vi "GetMessage.vi"(8 "entrée d'erreur":errorcluster caption="entrée d'erreur (pas d'erreur)", 11 "Message queue":refnum<queue>) -> (0 "sortie d'erreur":errorcluster, 1 "Data":variant, 2 "Message":string, 3 "Dup Message Queue":refnum<queue>)   [LabVIEW 2013, in "MessageQueues.lvlib"]
doc: "Ce VI permet la récupération d'un message en bas de pile, ainsi que sa donnée. Fonctionne en FIFO : First In First Out.\n\nEntrée :\nMessage queue : la pile concernée\nerror : entrée d'erreur\n\nSortie :\nDup Message Queue : Pile décrémenté\nMessage : Message récupéré en bas de pile\nData : Donnée lié au message du type variant.\nerro : sortie d'erreur."
uses:
  MessageQueues.lvlib
  Message Cluster.ctl
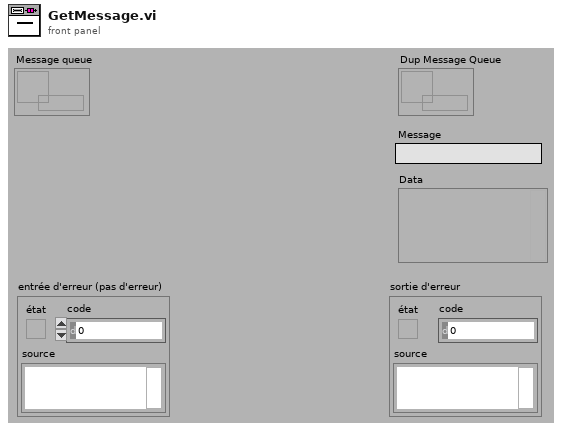
[diagram p1: front panel]
types:
  T1 = typedef "MessageQueues.lvlib/Message Cluster.ctl" = cluster{"Message":string, "Data":variant}
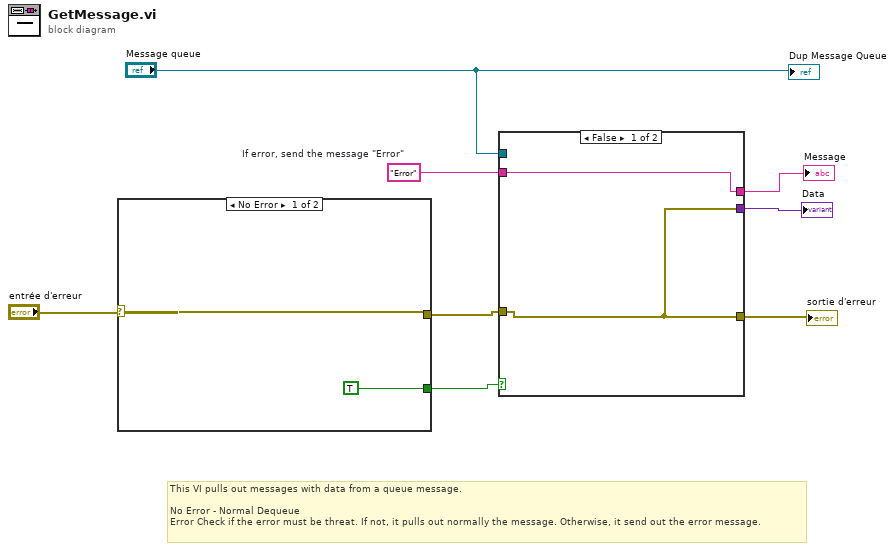
[diagram p0: block diagram]
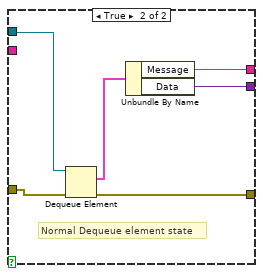
[diagram p2: hidden frame]
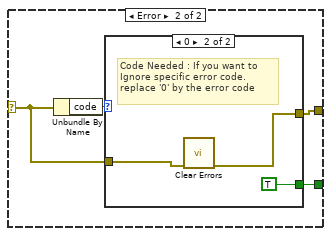
[diagram p3: hidden frame]
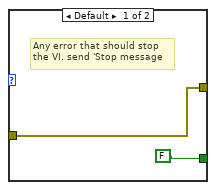
[diagram p4: hidden frame]
diagram:
  w5 = "Error"  # If error, send the message "Error"
  # "This VI pulls out messages with data from a queue message.\n\nNo Error - Normal Dequeue\nError Check if the error must be threat. If not, it pulls out normally the message. Otherwise, it send out the error message."
  n1 = case shown="No Error" "entrée d'erreur" {
    selector: "entrée d'erreur" -> [w9 w12]
    tunnel: [TRUE w14] -> w7
    tunnel: [w9 w11] -> w6
    frame No Error {
    }
    frame Error {
      n2 = Unbundle By Name(w12) -> ("code"=w13:i32)
      n3 = case shown="0" w13 {
        tunnel: [FALSE TRUE] -> w14
        tunnel: w12 -> [w15 w18]
        tunnel: [w15 w17] -> w11
        frame Default {
          # "Any error that should stop\nthe VI. send 'Stop message"
        }
        frame 0 {
          # "Code Needed : If you want to \nIgnore specific error code. \nreplace '0' by the error code"
          n4 = call <vilib>:"Clear Errors.vi"("error in (no error)"=w18) -> ("error out"=w17:errorcluster)  [unwired: 6 in]
        }
      }
    }
  }
  n5 = case shown="False" w7 {
    tunnel: "Message queue" -> [_ w27]
    tunnel: w6 -> [w20 w26]
    tunnel: w5 -> [w21 _]
    tunnel: [w20 w25] -> w4
    tunnel: [w21 w23] -> w2
    tunnel: [w20 w22] -> w1
    frame False {
    }
    frame True {
      # "Normal Dequeue element state"
      n6 = Dequeue Element(queue=w27, error in (no error)=w26) -> (element=w24:T1, error out=w25:errorcluster)  [unwired: 1 in, 2 out]
      n7 = Unbundle By Name(w24) -> ("Message"=w23:string, "Data"=w22:variant)
    }
  }
  "sortie d'erreur" <- w4
  "Message" <- w2
  "Data" <- w1
  "Dup Message Queue" <- "Message queue"
